vi "Caller.vi"(0 "Subtract in":refnum<class "Subtract.lvclass">, 2 "DVR In":refnum<data-value>, 11 "Error In":errorcluster) -> (4 "Subtract out":refnum<class "Subtract.lvclass">, 15 "Error Out":errorcluster)   [LabVIEW 2019, in "Subtract.lvclass"]
doc: "The VI opens the reference of operation UI that allows user to perform subtraction operation and runs the VI in the background."
uses:
  Subtract.lvclass
  Arithemtic Operation/Arithemetic Operation.lvclass
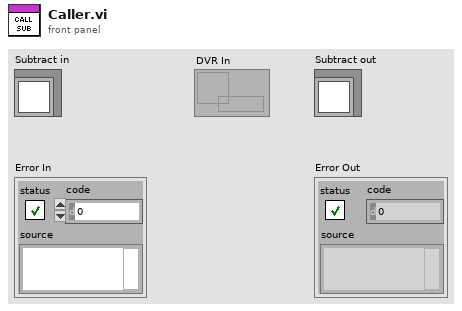
[diagram p1: front panel]
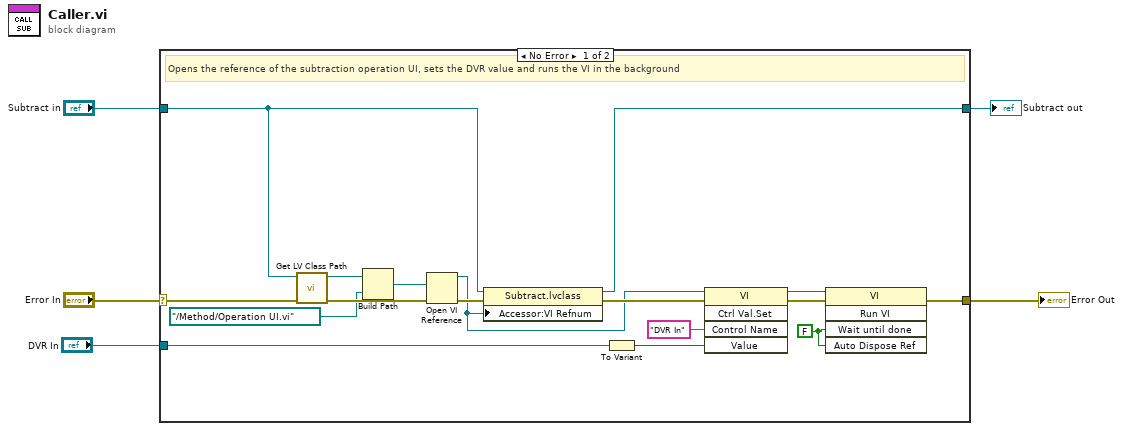
[diagram p0: block diagram]
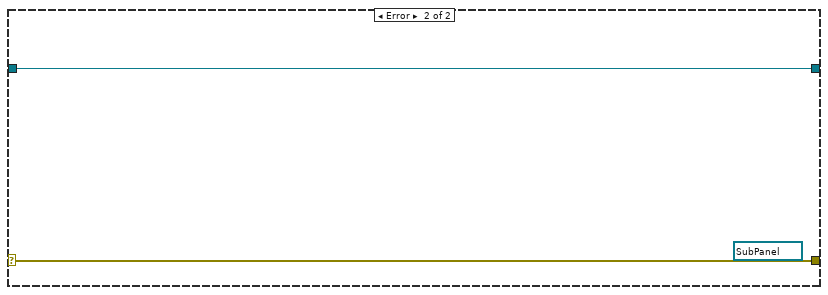
[diagram p2: hidden frame]
diagram:
  n1 = case shown="No Error" "Error In" {
    selector: "Error In" -> [w18 w24]
    tunnel: [w17 w23] -> w3
    tunnel: "Subtract in" -> [w16 w23]
    tunnel: "DVR In" -> [w8 _]
    tunnel: [w9 w24] -> w1
    frame No Error {
      w11 = FALSE ("Wait Until Done")
      # "Opens the reference of the subtraction operation UI, sets the DVR value and runs the VI in the background"
      n2 = call <vilib>:"Get LV Class Path.vi"("error in (no error)"=w18, "object"=w16) -> ("error out"=w22:errorcluster, "class path"=w21:path)  [unwired: 8 in]
      n3 = Build Path(base path=w21, name or relative path=path "../Method/Operation UI.vi") -> (appended path=w19:path)
      n4 = Open VI Reference(vi path=w19, error in (no error)=w22) -> (vi reference=w6:refnum<vi>, error out=w15:errorcluster)  [unwired: 4 in]
      n5 = property class="Subtract.lvclass"(reference=w16, error in=w15, "Accessor:VI Refnum"=w6) -> (reference out=w17:refnum<class "Subtract.lvclass">, error out=w10:errorcluster)
      n6 = To Variant(anything=w8) -> (Variant=w7:variant)
      n7 = invoke class="VI" method="Ctrl Val.Set"(reference=w6, error in=w10, "Control Name"="DVR In", "Value"=w7) -> (reference out=w13:refnum<vi>, error out=w12:errorcluster)  [unwired: 1 in, 3 out]
      n8 = invoke class="VI" method="Run VI"(reference=w13, error in=w12, "Wait until done"=w11, "Auto Dispose Ref"=w11) -> (error out=w9:errorcluster)  [unwired: 1 in, 4 out]
    }
    frame Error {
      (unwired) refnum<vi> refnum ("Sub Panel")
    }
  }
  "Error Out" <- w1
  "Subtract out" <- w3
